vi "Write Actor Filter.vi"(8 "error in (no error)":errorcluster, 10 "Actor Filter":T1={"PVMonitor"=FALSE, "PVProxy"=FALSE, "GUI"=FALSE, "Other"=TRUE}, 11 "CS++ObjectManager in":refnum<class "CS++ObjectManager.lvclass">) -> (0 "error out":errorcluster, 3 "CS++ObjectManager out":refnum<class "CS++ObjectManager.lvclass">)   [LabVIEW 2015, in "CS++ObjectManager.lvlib" / "CS++ObjectManager.lvclass"]
uses:
  CS++ObjectManager.lvclass
  CS++ObjectManager.lvclass/CS++ObjectManager.ctl
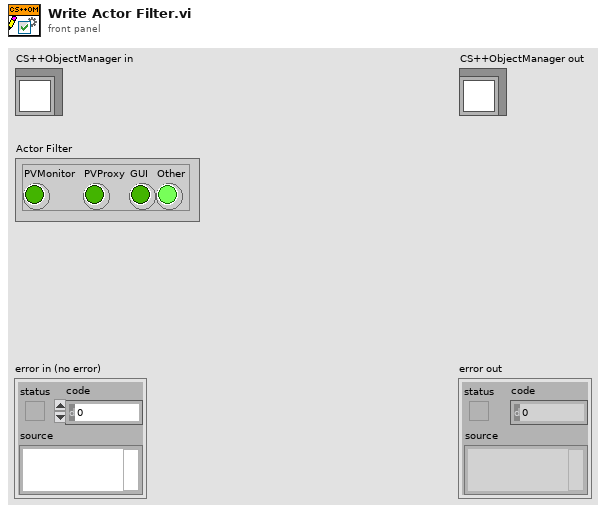
[diagram p1: front panel]
types:
  T1 = cluster{"PVMonitor":bool, "PVProxy":bool, "GUI":bool, "Other":bool}
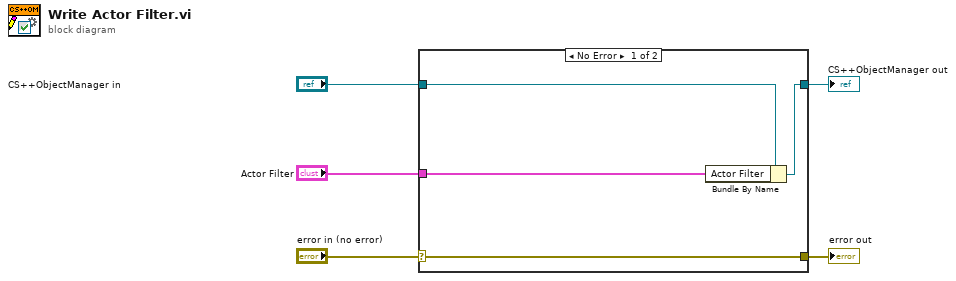
[diagram p0: block diagram]
diagram:
  n1 = case shown="No Error" "error in (no error)" {
    selector: "error in (no error)" -> [w9 w10]
    tunnel: [w9 w10] -> w4
    tunnel: [w7 w11] -> w2
    tunnel: "CS++ObjectManager in" -> [w8 w11]
    tunnel: "Actor Filter" -> [w6 _]
    frame No Error {
      n2 = Bundle By Name(cluster=w8, "Actor Filter"=w6) -> (w7:refnum<class "CS++ObjectManager.lvclass">)
    }
    frame Error {
    }
  }
  "error out" <- w4
  "CS++ObjectManager out" <- w2
